vi "Do.vi"(8 "error in (no error)":errorcluster, 10 "Actor in":refnum<class "Actor.lvclass">, 11 "Generate_no_B Msg":refnum<class "Generate_no_B Msg.lvclass">) -> (0 "error out":errorcluster, 2 "Actor out":refnum<class "Actor.lvclass">)   [LabVIEW 2025, in "Button_transfer.lvlib" / "Generate_no_B Msg.lvclass"]
doc: "This VI delivers the message to the actor by calling the appropriate method(s) on the actor."
uses:
  Generate_no_B Msg.lvclass
  Generate_no_B Msg.lvclass/Generate_no_B Msg.ctl
  C:/Users/halstead_rideriver/Documents/Labview_Practice/Tasks_Actor/B_Actor Messages/Random_B Msg/Random_B Msg.lvclass
  C:/Program Files (x86)/National Instruments/LabVIEW 2025/vi.lib/ActorFramework/Message/Message.lvclass
  C:/Users/halstead_rideriver/Documents/Labview_Practice/Tasks_Actor/Button_transfer Messages/Generate_no_B Msg/Generate_no_B Msg.lvclass
  34700b1e-4b1b-4205-ab4b-28631ba2a4c6.vi
  Button_transfer/Button_transfer.lvclass
  B_Actor Messages/Random_B Msg/Random_B Msg.lvclass
  <vilib>/ActorFramework/Actor/Actor.lvclass
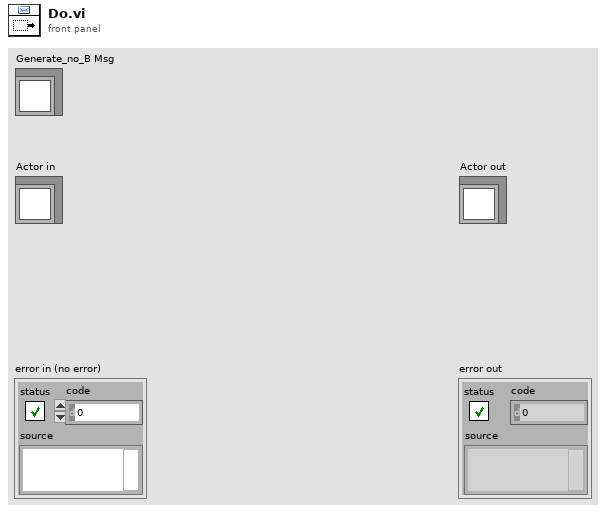
[diagram p1: front panel]
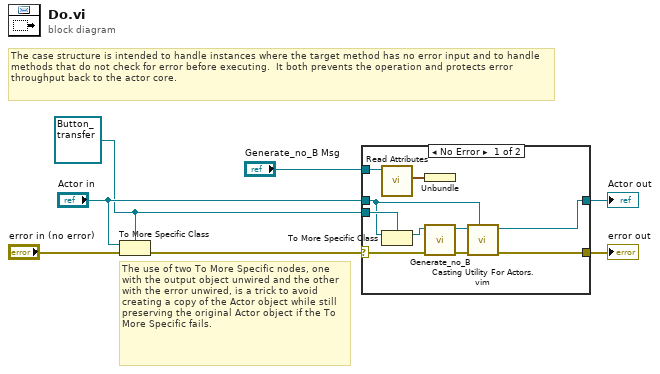
[diagram p0: block diagram]
diagram:
  w2 = refnum<class "Button_transfer.lvclass"> refnum ("Actor in")
  # "The use of two To More Specific nodes, one with the output object unwired and the other with the error unwired, is a trick to avoid creating a copy of the Actor object while still preserving the original Actor object if the To More Specific fails."
  # "The case structure is intended to handle instances where the target method has no error input and to handle methods that do not check for error before executing.  It both prevents the operation and protects error throughput back to the actor core."
  n1 = To More Specific Class(target class=w2, reference="Actor in", error in="error in (no error)") -> (error out=w6:errorcluster)  [unwired: 1 out]
  n2 = case shown="No Error" w6 {
    selector: w6 -> [w17 w19]
    tunnel: [w9 w19] -> w5
    tunnel: [w8 w18] -> w4
    tunnel: "Actor in" -> [w12 w18]
    tunnel: w2 -> [w13 _]
    tunnel: "Generate_no_B Msg" -> [w14 _]
    frame No Error {
      n3 = call "Read Attributes.vi"("Random_B Msg"=w14) -> ("Payload"=w15:cluster{"Random":u64})  [unwired: 10 in]
      n4 = To More Specific Class(target class=w13, reference=w12) -> (specific class reference=w16:refnum<class "Button_transfer.lvclass">)  [unwired: 1 in, 1 out]
      n5 = Unbundle(w15) -> ()  [unwired: 1 out]
      n6 = call-dynamic "Generate_no_B.vi"("error in (no error)"=w17, "Button_transfer in"=w16) -> ("error out"=w10:errorcluster, "Button_transfer out"=w11:refnum<class "Button_transfer.lvclass">)  [unwired: 8 in]
      n7 = call "Casting Utility For Actors.vim"("type"=w12, "error in (no error)"=w10, "Actor in"=w11) -> ("error out"=w9:errorcluster, "Actor out"=w8:refnum<class "Actor.lvclass">)  [unwired: 7 in]
    }
    frame Error {
      # "If type check fails, pass the original object out again."
    }
  }
  "error out" <- w5
  "Actor out" <- w4
